vi "Commit NIRFmx.vi"(8 "error in":errorcluster, 11 "PAE Reference In":T1) -> (0 "error out":errorcluster, 3 "PAE Reference Out":T1)   [LabVIEW 2023]
uses:
  <vilib>/niPAEML/Typedefs/Session Handle.ctl
  <vilib>/niPAEML/PAE Reference.lvclass
  <vilib>/niPAEML/PAE Reference.lvclass/PAE Reference.ctl
  <vilib>/niPAEML/Accessors/Read NI RFmx Session.vi
  <vilib>/niPAEML/Accessors/Read NI RFmx Port.vi
  <vilib>/niPAEML/Accessors/Read RBW (Hz).vi
  <vilib>/niPAEML/Accessors/Read Measurement Interval (s).vi
  <vilib>/niPAEML/Accessors/Read Expected Gain (dB).vi
  <vilib>/niPAEML/Accessors/Read Initial Power (dBm).vi
  <vilib>/niPAEML/Accessors/Read Rx Start Frequency (Hz).vi
  <vilib>/niPAEML/Accessors/Read RBW Filter Type.vi
  <vilib>/niPAEML/Accessors/Read RRC Alpha.vi
  <vilib>/niPAEML/Accessors/Read NI RFSG Session.vi
  <vilib>/niPAEML/Accessors/Read RFmx Reference Trigger Input Terminal.vi
  <vilib>/niPAEML/Accessors/Read RFSG Stimulus Mode.vi
  <vilib>/niPAEML/Accessors/Read RFSG to RFmx Trigger Routing Mode.vi
  <vilib>/niPAEML/Accessors/Read RFmx Reference Trigger Delay (s).vi
  <vilib>/niPAEML/Accessors/Read RFmx Reference Trigger Output Terminal.vi
  <vilib>/niPAEML/Accessors/Read RFmx to DCPower Trigger Routing Mode.vi
  <vilib>/niPAEML/Accessors/Write NI RFmx Session.vi
  <vilib>/RFmx/SpecAn/mx/RFmxSpecAn.llb/RFmxSpecAn Disable Trigger.vi
  <vilib>/RFmx/SpecAn/mx/RFmxSpecAn.llb/RFmxSpecAn Configure Digital Edge Trigger.vi
  <vilib>/niPAEML/PAE/PAEML.lvlib
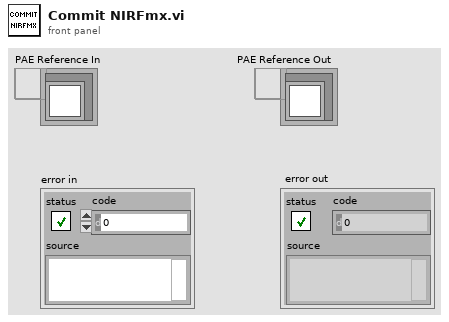
[diagram p1: front panel]
types:
  T1 = typedef "PAE Measurement.lvlib/PAE Reference.lvclass/Session Handle.ctl" = refnum<data-value>
  T2 = typedef "PAE Measurement.lvlib/PAE Reference.lvclass/RFmx Trigger Input Terminal.ctl" = string
  T3 = typedef "PAE Measurement.lvlib/PAE Reference.lvclass/RFSG Stimulus Mode.ctl" = enum16{"CW", "Pulsed CW"}
  T4 = typedef "PAE Measurement.lvlib/PAE Reference.lvclass/Trigger Routing Mode.ctl" = enum16{"Automatic", "Manual"}
  T5 = typedef "PAE Measurement.lvlib/PAE Reference.lvclass/RFmx Trigger Output Terminal.ctl" = string
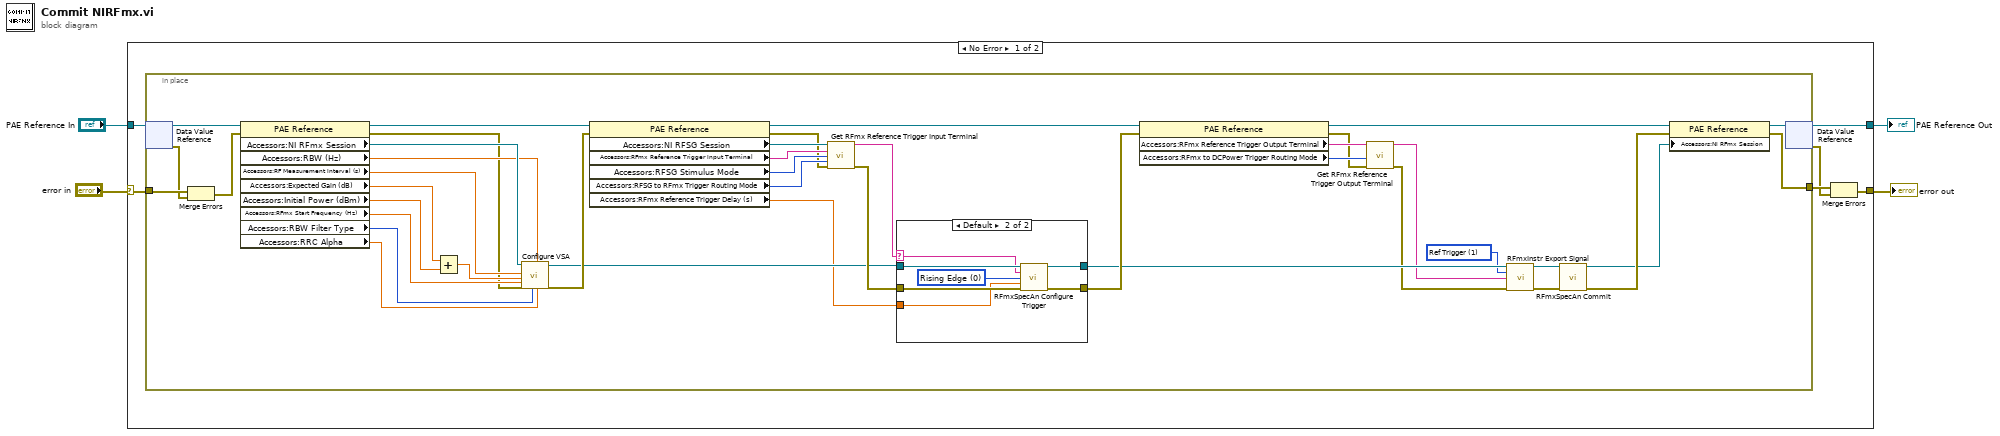
[diagram p0: block diagram]
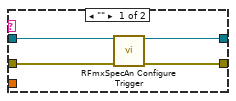
[diagram p2: hidden frame]
diagram:
  n1 = case shown="No Error" "error in" {
    selector: "error in" -> [w10 w64]
    tunnel: "PAE Reference In" -> [w6 w63]
    tunnel: [w5 w63] -> w1
    tunnel: [w7 w64] -> w3
    frame No Error {
      n2 = in-place {
        in-place-border: w10 -> [w51]
        in-place-border: [w48] -> w9
        w18 = 1 items=["Start Trigger", "Ref Trigger", "Advance Trigger", "Ready For Start Event", "Ready For Ref Event", "Ready For Advance Event", "End Of Record Event", "Done Event", "Reference Clock"] ("Export Signal Source")
        n3 = in-place-dvr #1(w6) -> (w46:refnum<class "PAE Reference.lvclass">, w50:errorcluster)
        n4 = Merge Errors(w51, w50) -> (w49:errorcluster)
        n5 = property class="PAE Reference"(reference=w46, error in=w49) -> (reference out=w38:refnum<class "PAE Reference.lvclass">, error out=w37:errorcluster, "Accessors:NI RFmx Session"=w47:refnum<k21>, "Accessors:RBW (Hz)"=w39:dbl, "Accessors:RF Measurement Interval (s)"=w44:dbl, "Accessors:Expected Gain (dB)"=w43:dbl, "Accessors:Initial Power (dBm)"=w42:dbl, "Accessors:RFmx Start Frequency (Hz)"=w40:dbl, "Accessors:RBW Filter Type"=w36:i32, "Accessors:RRC Alpha"=w35:dbl)
        n6 = Add(x=w43, y=w42) -> (x+y=w41:dbl)
        n7 = call "Configure VSA.vi"("instrument handle in"=w47, "measurement interval (s)"=w44, "reference level"=w41, "carrier frequency"=w40, "error in"=w37, "RBW Filter Type"=w36, "RBW (Hz)"=w39, "RRC Alpha"=w35) -> ("instrument handle out"=w27:refnum<k21>, "error out"=w34:errorcluster)  [unwired: 10 in]
        n8 = property class="PAE Reference"(reference=w38, error in=w34) -> (reference out=w24:refnum<class "PAE Reference.lvclass">, error out=w29:errorcluster, "Accessors:NI RFSG Session"=w33:refnum<k15>, "Accessors:RFmx Reference Trigger Input Terminal"=w32:T2, "Accessors:RFSG Stimulus Mode"=w31:T3, "Accessors:RFSG to RFmx Trigger Routing Mode"=w30:T4, "Accessors:RFmx Reference Trigger Delay (s)"=w25:dbl)
        n9 = call <vilib>:"Get RFmx Reference Trigger Input Terminal.vi"("RFSG Instrument Handle"=w33, "User Specified RFmx Reference Trigger Input Terminal"=w32, "RFSG Stimulus Mode"=w31, "RFSG to RFmx Trigger Routing Mode"=w30, "error in"=w29) -> ("RFmx Reference Trigger Input Terminal"=w26:T2, "error out"=w28:errorcluster)  [unwired: 9 in]
        n10 = case shown="Default" w26 {
          selector: w26 -> [_ w60]
          tunnel: w28 -> [w55 w62]
          tunnel: w27 -> [w53 w61]
          tunnel: w25 -> [_ w58]
          tunnel: [w54 w57] -> w23
          tunnel: [w52 w56] -> w19
          frame "" {
            n11 = call-poly <vilib>:"RFmxSpecAn Configure Trigger.vi"("Instrument Handle In"=w53, "error in (no error)"=w55) -> ("Instrument Handle Out"=w52:refnum<k21>, "error out"=w54:errorcluster)  [unwired: 12 in]
          }
          frame Default {
            w59 = 0 items=["Rising Edge", "Falling Edge"] ("Digital Edge")
            n12 = call-poly <vilib>:"RFmxSpecAn Configure Trigger.vi"("Instrument Handle In"=w61, "Digital Edge Source"=w60, "Digital Edge"=w59, "Trigger Delay (s)"=w58, "error in (no error)"=w62) -> ("Instrument Handle Out"=w56:refnum<k21>, "error out"=w57:errorcluster)  [unwired: 9 in]
          }
        }
        n13 = property class="PAE Reference"(reference=w24, error in=w23) -> (reference out=w15:refnum<class "PAE Reference.lvclass">, error out=w20:errorcluster, "Accessors:RFmx Reference Trigger Output Terminal"=w22:T5, "Accessors:RFmx to DCPower Trigger Routing Mode"=w21:T4)
        n14 = call <vilib>:"Get RFmx Reference Trigger Output Terminal.vi"("User Specified RFmx ReferenceTrigger Output Terminal"=w22, "RFmx to DCPower Trigger Routing Mode"=w21, "error in"=w20) -> ("RFmx ReferenceTrigger Output Terminal"=w17:T5, "error out"=w16:errorcluster)  [unwired: 11 in]
        n15 = call <vilib>:"RFmxInstr Export Signal.vi"("Instrument Handle In"=w19, "Export Signal Source"=w18, "Export Signal Output Terminal"=w17, "error in (no error)"=w16) -> ("Instrument Handle Out"=w13:refnum<k21>, "error out"=w14:errorcluster)  [unwired: 10 in]
        n16 = call <vilib>:"RFmxSpecAn Commit.vi"("Instrument Handle In"=w13, "error in (no error)"=w14) -> ("Instrument Handle Out"=w11:refnum<k21>, "error out"=w12:errorcluster)  [unwired: 12 in]
        n17 = property class="PAE Reference"(reference=w15, error in=w12, "Accessors:NI RFmx Session"=w11) -> (reference out=w45:refnum<class "PAE Reference.lvclass">, error out=w48:errorcluster)
        n18 = in-place-dvr #1(w45) -> (w5:T1, w8:errorcluster)
      }
      n19 = Merge Errors(w9, w8) -> (w7:errorcluster)
    }
    frame Error {
    }
  }
  "PAE Reference Out" <- w1
  "error out" <- w3
